vi "Basic Power Measurement (DAQmx).vi"() -> ()   [LabVIEW 2024]
doc: "Demonstrates how to implement basic power measurement on a three-phase electrical power system, such as power and energy values, frequency amplitudes, and symmetrical components."
uses:
  <vilib>/Utility/error.llb/DialogType.ctl
  <vilib>/DAQmx/read.llb/DAQmx Read (Analog 1D Wfm NChan NSamp).vi
  <vilib>/addons/Electrical Power/Basic/Measurement/RMS (N Channels).vi
  <vilib>/addons/Electrical Power/Basic/Measurement/RMS (1 Channel).vi
  <vilib>/Analysis/5stat.llb/RMS (DBL).vi
  <vilib>/DAQmx/create/channels.llb/DAQmx Create Channel (AI-Voltage-Basic).vi
  <vilib>/DAQmx/create/channels.llb/DAQmx Create Channel (AI-Current-Basic).vi
  <vilib>/DAQmx/configure/timing.llb/DAQmx Timing (Sample Clock).vi
  <vilib>/DAQmx/miscellaneous.llb/DAQmx Fill In Error Info.vi
  <vilib>/addons/Electrical Power/Basic/Measurement/Frequency (N Channels).vi
  <vilib>/measure/maUtilsandCtls.llb/ma_Check Waveform Timing.vi
  <vilib>/addons/Electrical Power/Basic/Measurement/Fundamental Vector (N Channels).vi
  <vilib>/addons/Electrical Power/Basic/Measurement/Power (N Channels).vi
  <vilib>/addons/Electrical Power/Basic/Measurement/Energy (N Channels).vi
  <vilib>/addons/Electrical Power/Basic/NI_EP_Basic.lvlib
  <resource>/objmgr/daqmx.rc
panel:
  in  "Tab Control":T1(tab)
  in  "voltage channels":tag="voltage-input/ai0, voltage-input/ai2:1"
  in  "current channels":tag="current-input/ai0, current-input/ai2:1"
  in  "maximum voltage value":dbl=300.0 caption="Maximum Value" format="%0.2f"
  in  "minimum voltage value":dbl=-300.0 caption="Minimum Value" format="%0.2f"
  in  "maximum current value":dbl=0.002 format="%0.3f"
  in  "minimum current value":dbl=-0.002 format="%0.3f"
  in  "number of samples per channel":i32=10000
  in  "DAQmx sample rate [Hz]":dbl=50000.0 format="%0.2f"
  out "Voltage Waveforms":waveform(dbl)[](graph)
  out "Current Waveforms":waveform(dbl)[](graph)
  out "frequency [Hz]":dbl
  out "voltage RMS values":dbl[](array[numeric])
  out "current RMS values":dbl[](array[numeric])
  out "energy values":T2(array[cluster])
  out "power values":T3(array[cluster])
  out "voltage fundamental vectors":cdb[](array[numeric])
  out "current fundamental vectors":cdb[](array[numeric])
  out "zero sequence":cdb
  out "positive sequence":cdb
  out "negative sequence":cdb
  out "Voltage Vector Diagram":dbl[](graph)
  in  "stop":bool
  # "Overview: Demonstrates how to implement basic power measurement on a three-phase electrical power system.\nRequirements: NI-DAQmx, Electrical Power Toolkit Base Edition\nInstructions: 1. Connect the signals you want to perform basic power measurement to the DAQ devices.\n                        2. Configure Settings and run this VI."
  # "Channel Scaling Info"
  # "Sampling Info"
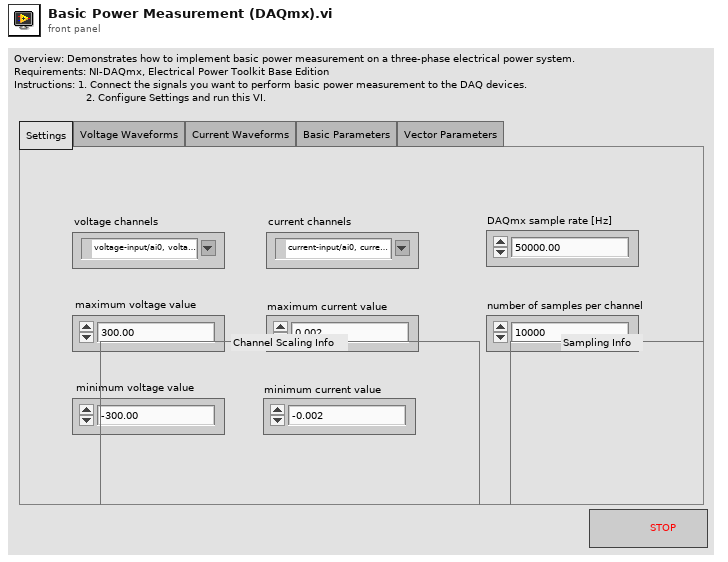
[diagram p1: front panel]
types:
  T1 = enum32{"Settings", "Voltage Waveforms", "Current Waveforms", "Basic Parameters", "Vector Parameters"}
  T2 = cluster{"active energy [Wh]":dbl, "apparent energy [VAh]":dbl, "reactive energy [VARh]":dbl}[]
  T3 = cluster{"active power [W]":dbl, "apparent power [VA]":dbl, "reactive power [VAR]":dbl, "power factor":dbl}[]
  T4 = typedef "DialogType.ctl" = u16
  T5 = typedef "NI_EP_Basic.lvlib/basic_Power Value.ctl" = cluster{"active power [W]":dbl, "apparent power [VA]":dbl, "reactive power [VAR]":dbl, "power factor":dbl}
  T6 = typedef "NI_EP_Basic.lvlib/basic_Energy Value.ctl" = cluster{"active energy [Wh]":dbl, "apparent energy [VAh]":dbl, "reactive energy [VARh]":dbl}
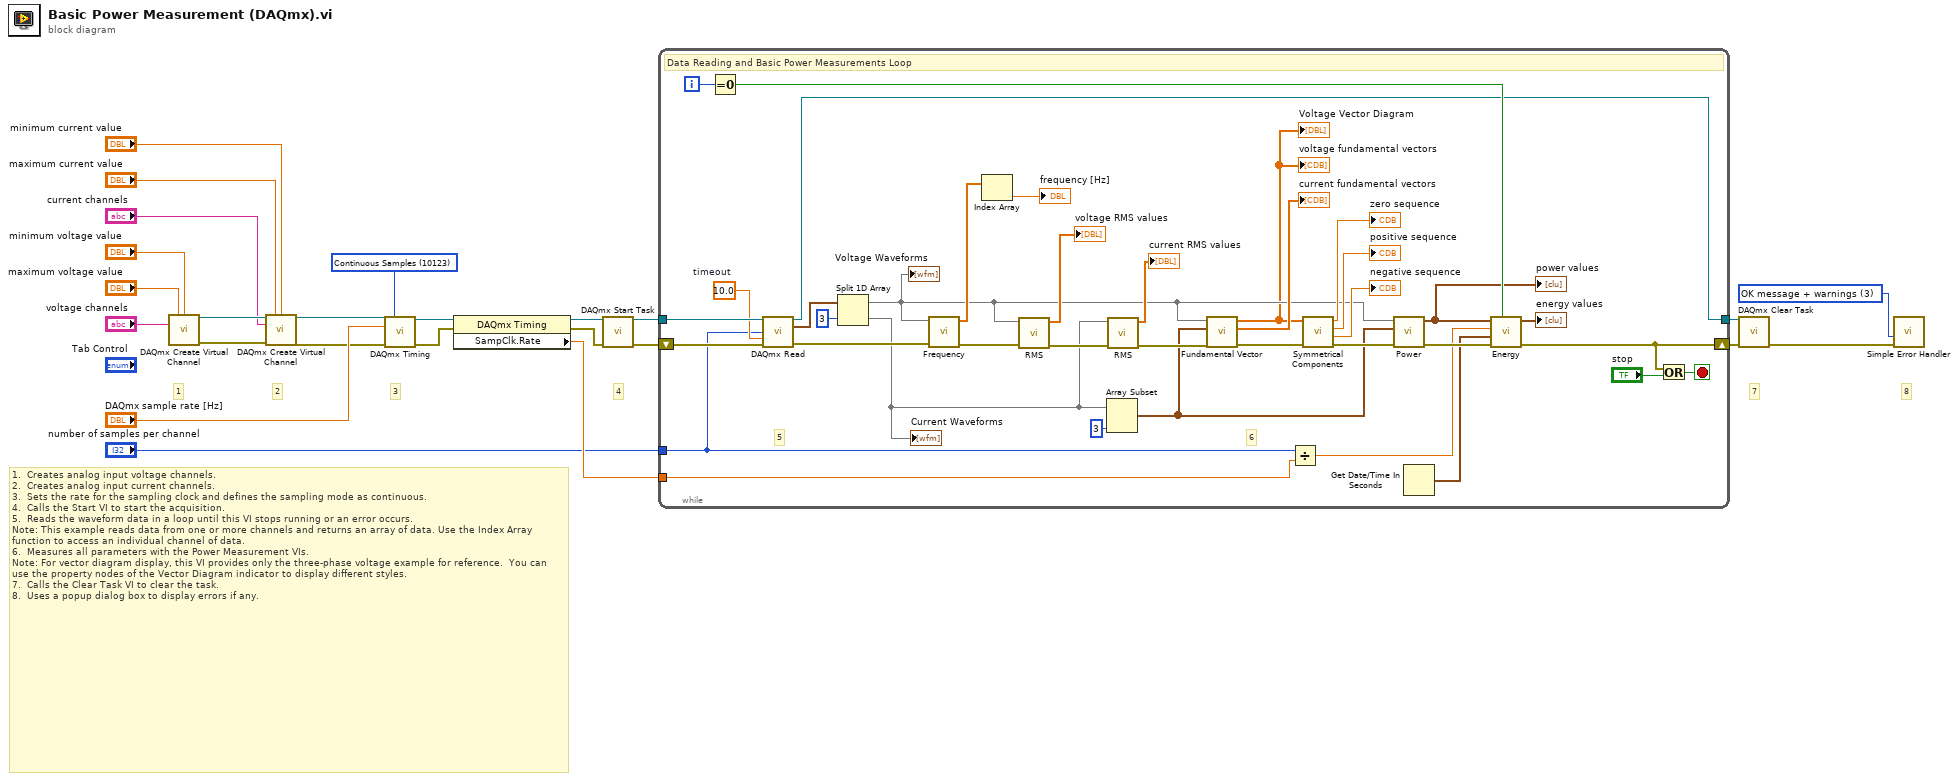
[diagram p0: block diagram]
diagram:
  w18 = T4 3 items=["no dialog", "OK message", "continue or stop message", "OK message + warnings", "continue/stop + warnings"] ("type of dialog (OK msg:1)")
  w19 = 10123 items=["Finite Samples"=10178, "Continuous Samples"=10123] ("sample mode")
  # "1.  Creates analog input voltage channels.\n2.  Creates analog input current channels.\n3.  Sets the rate for the sampling clock and defines the sampling mode as continuous.\n4.  Calls the Start VI to start the acquisition.\n5.  Reads the waveform data in a loop until this VI stops running or an error occurs.\nNote: This example reads data from one or more channels and returns an array of data. Use the Index Array function to access an individual channel of data.\n6.  Measures all parameters with the Power Measurement VIs.\nNote: For vector diagram display, this VI provides only the three-phase voltage example for reference.  You can use the property nodes of the Vector Diagram indicator to display different styles.\n7.  Calls the Clear Task VI to clear the task.\n8.  Uses a popup dialog box to display errors if any."
  # "8"
  # "7"
  # "4"
  # "3"
  # "2"
  # "1"
  n1 = call-poly <vilib>:"DAQmx Create Virtual Channel.vi"("maximum value"="maximum voltage value", "minimum value"="minimum voltage value", "physical channels"="voltage channels") -> ("task out"=w15:refnum<k21>, "error out"=w14:errorcluster)  [unwired: 11 in]
  n2 = call-poly <vilib>:"DAQmx Create Virtual Channel.vi"("task in"=w15, "maximum value"="maximum current value", "minimum value"="minimum current value", "physical channels"="current channels", "error in"=w14) -> ("task out"=w13:refnum<k21>, "error out"=w12:errorcluster)  [unwired: 9 in]
  n3 = call-poly <vilib>:"DAQmx Timing.vi"("task/channels in"=w13, "sample mode"=w19, "rate"="DAQmx sample rate [Hz]", "error in"=w12) -> ("task out"=w6:refnum<k21>, "error out"=w4:errorcluster)  [unwired: 10 in]
  n4 = property class="DAQmx Timing"(reference=w6, error in=w4) -> (reference out=w5:refnum<k21>, error out=w3:errorcluster, "SampClk.Rate"=w2:dbl)
  n5 = call <vilib>:"DAQmx Start Task.vi"("task/channels in"=w5, "error in"=w3) -> ("task out"=w21:refnum<k21>, "error out"=w8:errorcluster)  [unwired: 12 in]
  n6 = while {
    tunnel: w21 -> [w61]
    tunnel: [w36] -> w20
    shift-right: [w26] -> w16
    shift-left: w8 -> [w41]
    tunnel: w2 -> [w51]
    tunnel: "number of samples per channel" -> [w27]
    i -> [w53]
    stop <- w60 stop-if-true
    w29 = 10.0  # timeout
    # "6"
    # "5"
    # "Data Reading and Basic Power Measurements Loop"
    n7 = Equal To 0?(x=w53) -> (x = 0?=w52:bool)
    n8 = call-poly <vilib>:"DAQmx Read.vi"("task/channels in"=w61, "number of samples per channel"=w27, "timeout"=w29, "error in"=w41) -> ("task out"=w36:refnum<k21>, "data"=w49:waveform(dbl)[], "error out"=w40:errorcluster)  [unwired: 9 in]
    n9 = Split 1D Array(array=w49, index=3) -> (first subarray=w28:waveform(dbl)[], second subarray=w30:waveform(dbl)[])
    "Voltage Waveforms" <- w28
    "Current Waveforms" <- w30
    n10 = call-poly <vilib>:"Frequency.vi"("error in (no error)"=w40, "waveforms"=w28) -> ("error out"=w59:errorcluster, "frequencies"=w58:dbl[])  [unwired: 8 in]
    n11 = Index Array(array=w58) -> (element=→"frequency [Hz]":dbl)  [unwired: 1 in]
    n12 = call-poly <vilib>:"RMS.vi"("error in (no error)"=w59, "waveforms"=w28) -> ("error out"=w47:errorcluster, "RMS values"=→"voltage RMS values":dbl[])  [unwired: 8 in]
    n13 = Array Subset(array=w30, length=3) -> (w34:waveform(dbl)[])  [unwired: 1 in]
    n14 = call-poly <vilib>:"RMS.vi"("error in (no error)"=w47, "waveforms"=w30) -> ("error out"=w46:errorcluster, "RMS values"=→"current RMS values":dbl[])  [unwired: 8 in]
    n15 = call-poly <vilib>:"Fundamental Vector.vi"("error in (no error)"=w46, "current waveforms"=w34, "voltage waveforms"=w28) -> ("error out"=w55:errorcluster, "current fundamental vectors"=→"current fundamental vectors":cdb[], "voltage fundamental vectors"=w25:cdb[])  [unwired: 5 in, 1 out]
    "Voltage Vector Diagram" <- w25
    "voltage fundamental vectors" <- w25
    n16 = Divide(x=w27, y=w51) -> (x/y=w50:dbl)
    n17 = call <vilib>:"Symmetrical Components.vi"("error in (no error)"=w55, "3-phase phasors"=w25) -> ("error out"=w54:errorcluster, "negative sequence"=→"negative sequence":cdb, "positive sequence"=→"positive sequence":cdb, "zero sequence"=→"zero sequence":cdb)  [unwired: 6 in]
    n18 = call-poly <vilib>:"Power.vi"("error in (no error)"=w54, "current waveforms"=w34, "voltage waveforms"=w28) -> ("error out"=w57:errorcluster, "power values"=w33:T5[])  [unwired: 7 in]
    "power values" <- w33
    n19 = Get Date/Time In Seconds() -> (seconds since 1Jan1904=w56:timestamp)
    n20 = call-poly <vilib>:"Energy.vi"("reset? (F)"=w52, "error in (no error)"=w57, "start timestamp"=w56, "interval length [s]"=w50, "power values"=w33) -> ("error out"=w26:errorcluster, "energy values"=→"energy values":T6[])  [unwired: 4 in, 1 out]
    n21 = Or(x=w26, y="stop") -> (x .or. y?=w60:bool)
  }
  n22 = call <vilib>:"DAQmx Clear Task.vi"("task in"=w20, "error in"=w16) -> ("error out"=w22:errorcluster)  [unwired: 13 in]
  n23 = call <vilib>:"Simple Error Handler.vi"("type of dialog (OK msg:1)"=w18, "error in (no error)"=w22) -> ()  [unwired: 3 in, 5 out]
